vi "calc_repeller_delay_T0.vi"(0 "Variable Values Out":T1, 7 "Trap Delay Array":dbl[](array[numeric])) -> (8 "Total Repeller Delay / us":dbl)   [LabVIEW 2023]
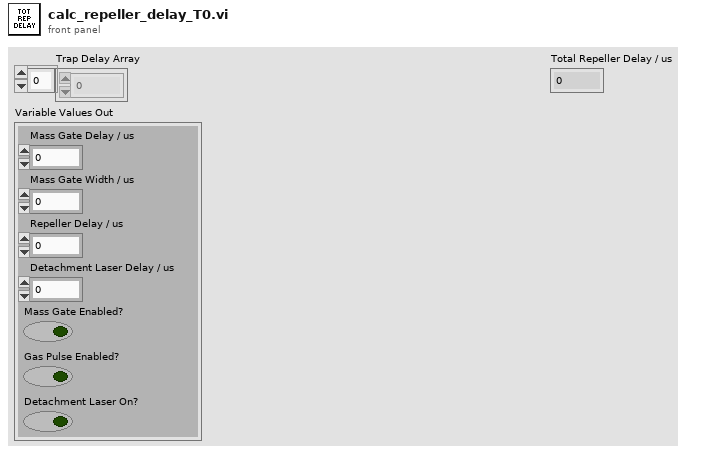
[diagram p1: front panel]
types:
  T1 = cluster{"Mass Gate Delay / us":dbl, "Mass Gate Width / us":dbl, "Repeller Delay / us":dbl, "Detachment Laser Delay / us":dbl, "Mass Gate Enabled?":bool, "Gas Pulse Enabled?":bool, "Detachment Laser On?":bool}
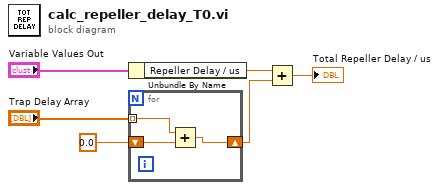
[diagram p0: block diagram]
diagram:
  n1 = Unbundle By Name("Variable Values Out") -> ("Repeller Delay / us"=w3:dbl)
  n2 = for {
    tunnel: "Trap Delay Array" -> [w7] mode=indexing
    shift-right: [w8] -> w2
    shift-left: 0.0 -> [w9]
    n3 = Add(x=w7, y=w9) -> (x+y=w8:dbl)
  }
  n4 = Add(x=w3, y=w2) -> (x+y=→"Total Repeller Delay / us":dbl)
